vi "Take Line Image.vi"(6 "Image Name":string="composite image", 7 "Quality":enum16{"perfect", "medium", "low"}(ring), 8 "error in":errorcluster, 9 "Line End":refnum<class "Vec3d Class.lvclass">, 10 "Line Start":refnum<class "Vec3d Class.lvclass">, 11 "CameraTool in":refnum<class "CameraTool Class.lvclass">) -> (0 "error out":errorcluster, 2 "Physical Image":T1, 3 "CameraTool out":refnum<class "CameraTool Class.lvclass">)   [LabVIEW 2011, in "CameraTool Class.lvclass"]
uses:
  CameraTool Class.lvclass
  Vec3d Class/Vec3d Class.lvclass
  Utils/Type Definitions/Physical Image.ctl
  <vilib>/vision/Image Controls.llb/IMAQ Image.ctl
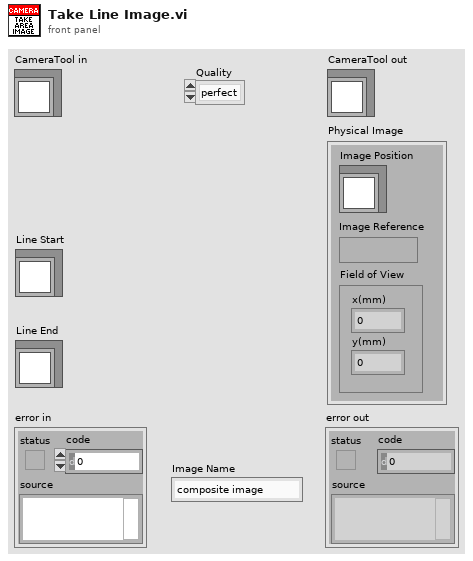
[diagram p1: front panel]
types:
  T1 = typedef "Physical Image.ctl" = cluster{"Image Position":refnum<class "Vec3d Class.lvclass">, "Image Reference":T2, "Field of View":cluster{"x(mm)":dbl, "y(mm)":dbl}}
  T2 = typedef "IMAQ Image.ctl" = refnum<image>
  T3 = typedef "Gantry_Camera.ctl" = cluster{"Name":string, "IMAQ Session":T4, "Group":u32, "Open?":bool, "Interface Name":string, "Field of View":cluster{"x-mm":dbl, "y-mm":dbl}}
  T4 = typedef "IMAQdx.ctl" = refnum<k21>
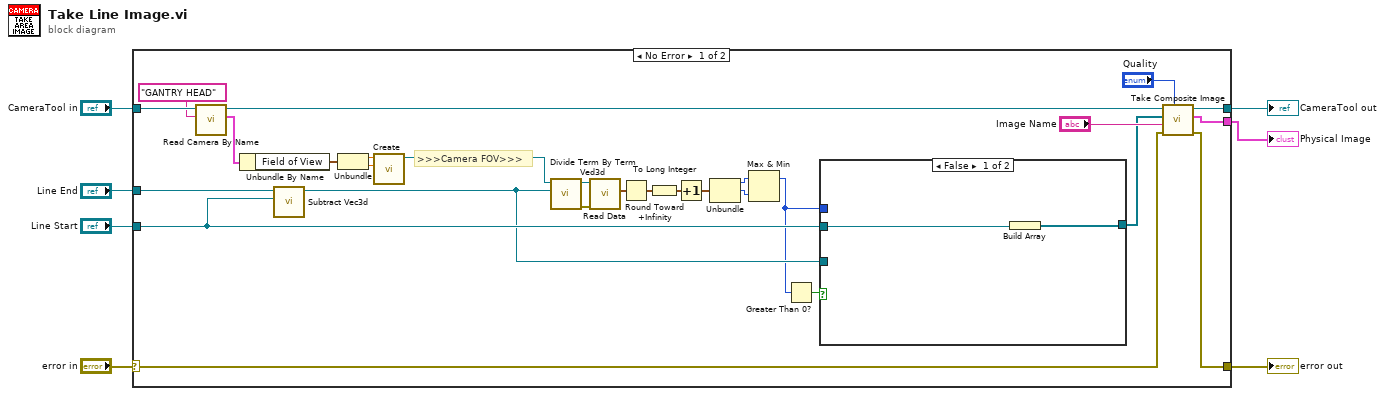
[diagram p0: block diagram]
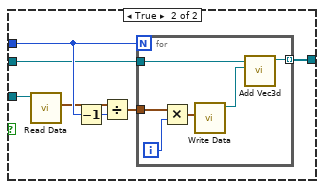
[diagram p2: hidden frame]
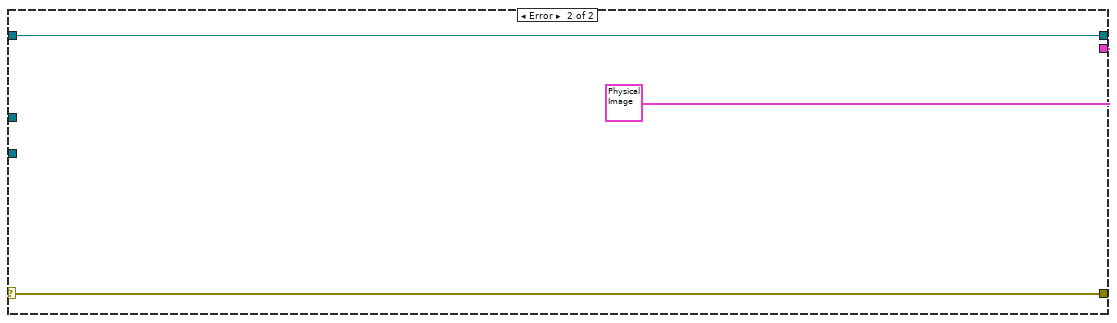
[diagram p3: hidden frame]
diagram:
  n1 = case shown="No Error" "error in" {
    selector: "error in" -> [w23 w53]
    tunnel: [w22 w53] -> w6
    tunnel: [w24 w52] -> w4
    tunnel: "CameraTool in" -> [w35 w52]
    tunnel: "Line End" -> [w18 _]
    tunnel: "Line Start" -> [w12 _]
    tunnel: [w21 T1 {"Image Position"=refnum, "Image Reference"=refnum, "Field of View"={"x(mm)"=0.0, "y(mm)"=0.0}} ("Physical Image")] -> w2
    frame No Error {
      # ">>>Camera FOV>>>"
      n2 = call-dynamic "Read Camera By Name.vi"("Camera Name"="GANTRY HEAD", "Gantry in"=w35) -> ("Camera"=w33:T3, "Gantry out"=w25:refnum<class "CameraTool Class.lvclass">)  [unwired: 7 in, 1 out]
      n3 = Unbundle By Name(w33) -> ("Field of View"=w30:cluster{"x-mm":dbl, "y-mm":dbl})
      n4 = call "Subtract Vec3d.vi"("Vec3d in 2"=w12, "Vec3d in 1"=w18) -> ("Vec3d Class out"=w11:refnum<class "Vec3d Class.lvclass">)  [unwired: 8 in, 1 out]
      n5 = Unbundle(w30) -> ("x-mm"=w32:dbl, "y-mm"=w31:dbl)
      n6 = call "Create.vi"("Y"=w31, "X"=w32) -> ("Vec3d Class out"=w26:refnum<class "Vec3d Class.lvclass">)  [unwired: 8 in, 1 out]
      n7 = call-dynamic "Divide Term By Term Ved3d.vi"("Vec3d in 2"=w11, "Vec3d in 1"=w26) -> ("error out"=w29:errorcluster, "Vec3d Class out"=w28:refnum<class "Vec3d Class.lvclass">)  [unwired: 8 in]
      n8 = call-dynamic "Read Data.vi"("error in (no error)"=w29, "Vec3d Class in"=w28) -> ("Data"=w27:cluster{"X":dbl, "Y":dbl, "Z":dbl})  [unwired: 7 in, 2 out]
      n9 = Round Toward +Infinity(x=w27) -> (ceil(x): smallest int >= x=w17:cluster{"X":dbl, "Y":dbl, "Z":dbl})
      n10 = To Long Integer(number=w17) -> (32bit integer=w16:cluster{"X":i32, "Y":i32, "Z":i32})
      n11 = Increment(x=w16) -> (x+1=w15:cluster{"X":i32, "Y":i32, "Z":i32})
      n12 = Unbundle(w15) -> ("X"=w14:i32, "Y"=w13:i32)  [unwired: 1 out]
      n13 = Max & Min(x=w14, y=w13) -> (max(x,y)=w9:i32)  [unwired: 1 out]
      n14 = Greater Than 0?(x=w9) -> (x > 0?=w10:bool)
      n15 = case shown="False" w10 {
        tunnel: [w36 w44] -> w8
        tunnel: w9 -> [_ w43]
        tunnel: w12 -> [w37 w41]
        tunnel: w11 -> [_ w40]
        frame False {
          n16 = Build Array(w37) -> (w36:refnum<class "Vec3d Class.lvclass">[])
        }
        frame True {
          n17 = call-dynamic "Read Data.vi"("Vec3d Class in"=w40) -> ("Data"=w39:cluster{"X":dbl, "Y":dbl, "Z":dbl})  [unwired: 8 in, 2 out]
          n18 = Decrement(x=w43) -> (x-1=w42:i32)
          n19 = Divide(x=w39, y=w42) -> (x/y=w38:cluster{"X":dbl, "Y":dbl, "Z":dbl})
          n20 = for {
            N: w43 -> [_]
            tunnel: [w50] -> w44 mode=indexing
            tunnel: w41 -> [w49]
            tunnel: w38 -> [w47]
            i -> [w46]
            n21 = Multiply(x=w47, y=w46) -> (x*y=w45:cluster{"X":dbl, "Y":dbl, "Z":dbl})
            n22 = call "Write Data.vi"("Data"=w45) -> ("Vec3d Class out"=w48:refnum<class "Vec3d Class.lvclass">)  [unwired: 9 in, 1 out]
            n23 = call-dynamic "Add Vec3d.vi"(10:"Vec3d Class in"=w48, 11:"Vec3d Class in"=w49) -> ("Vec3d Class out"=w50:refnum<class "Vec3d Class.lvclass">)  [unwired: 8 in, 1 out]
          }
        }
      }
      n24 = call "Take Composite Image.vi"("Quality"="Quality", "error in"=w23, "Image Name"="Image Name", "Points"=w8, "CameraTool in"=w25) -> ("error out"=w22:errorcluster, "Physical Image"=w21:T1, "CameraTool out"=w24:refnum<class "CameraTool Class.lvclass">)  [unwired: 4 in]
    }
    frame Error {
    }
  }
  "error out" <- w6
  "CameraTool out" <- w4
  "Physical Image" <- w2
